vi "GEN40-38-LAN Send Voltage Setting.vi"(8 "error in (no error)":errorcluster, 11 "GEN40-38-LAN in":refnum<class "GEN40-38-LAN.lvclass">) -> (0 "error out":errorcluster, 3 "GEN40-38-LAN out":refnum<class "GEN40-38-LAN.lvclass">)   [LabVIEW 2018, in "GEN40-38-LAN.lvlib" / "GEN40-38-LAN.lvclass"]
doc: "This VI is used to send the Voltage Setting to the Power Supply."
uses:
  GEN40-38-LAN.lvclass
  PPLs/Power Supply/Parent/Power_Supply.lvlibp/Power Supply.lvclass
  C:/Projects/LabVIEW/PPLs/Power Supply/Parent/Power_Supply.lvlibp/Power Supply.lvclass
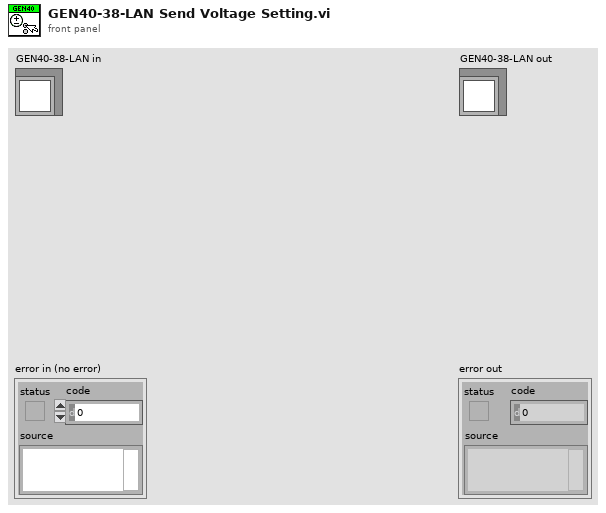
[diagram p1: front panel]
types:
  T1 = typedef "Power_Supply.lvlibp/Supply Settings.ctl" = cluster{"Voltage":dbl, "Current":dbl, "Output":bool}
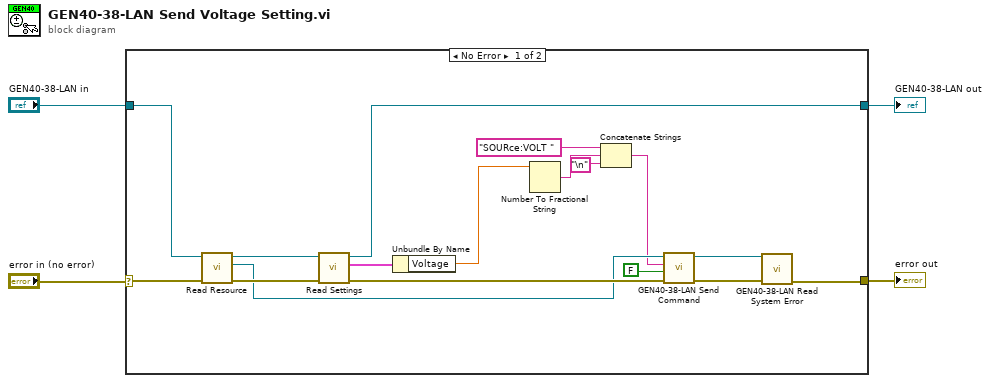
[diagram p0: block diagram]
diagram:
  n1 = case shown="No Error" "error in (no error)" {
    selector: "error in (no error)" -> [w5 w23]
    tunnel: [w7 w23] -> w3
    tunnel: [w10 w22] -> w1
    tunnel: "GEN40-38-LAN in" -> [w6 w22]
    frame No Error {
      n2 = call "Read Resource.vi"("error in"=w5, "Power Supply in"=w6) -> ("error out"=w21:errorcluster, "Resource"=w17:refnum<visa-resource-name>, "Power Supply out"=w20:refnum<class "GEN40-38-LAN.lvclass">)  [unwired: 7 in]
      n3 = call "Read Settings.vi"("error in (no error)"=w21, "Power Supply in"=w20) -> ("error out"=w18:errorcluster, "Settings"=w19:T1, "Power Supply out"=w10:refnum<class "GEN40-38-LAN.lvclass">)  [unwired: 7 in]
      n4 = Unbundle By Name(w19) -> ("Voltage"=w16:dbl)
      n5 = Number To Fractional String(number=w16) -> (F-format string=w14:string)  [unwired: 3 in]
      n6 = Concatenate Strings("SOURce:VOLT ", w14, "\n" ("string")) -> (w12:string)
      n7 = call "GEN40-38-LAN Send Command.vi"("error in (no error)"=w18, "Wait for Response?"=FALSE, "Command"=w12, "VISA resource name"=w17) -> ("error out"=w9:errorcluster, "VISA resource name out"=w8:refnum<visa-resource-name>)  [unwired: 5 in, 1 out]
      n8 = call "GEN40-38-LAN Read System Error.vi"("error in (no error)"=w9, "Resource"=w8) -> ("error out"=w7:errorcluster)  [unwired: 9 in]
    }
    frame Error {
    }
  }
  "error out" <- w3
  "GEN40-38-LAN out" <- w1
